vi "lab#5 (for loop).vi"() -> ()   [LabVIEW 2016]
panel:
  out "Elapsed Time (s)":dbl
  out "millisecond timer value":u32
  out "Time has Elapsed":bool
  out "number (0 to 1)":dbl
  out "Numeric 2":i32
  in  "Numeric":i32
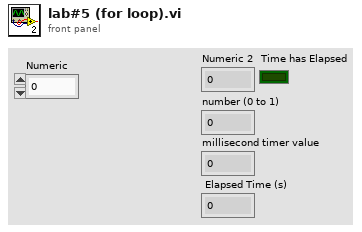
[diagram p1: front panel]
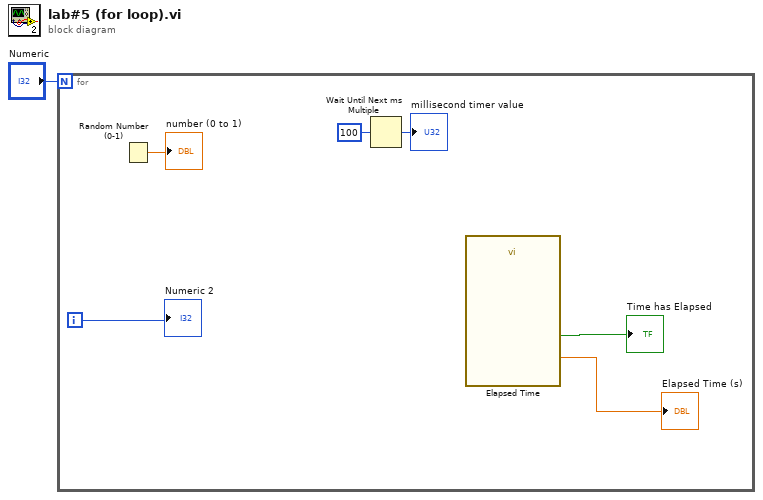
[diagram p0: block diagram]
diagram:
  n1 = for {
    N: "Numeric" -> [_]
    i -> [w7]
    n2 = Random Number (0-1)() -> (number: 0 to 1=→"number (0 to 1)":dbl)
    n3 = Wait Until Next ms Multiple(millisecond multiple=u32 100) -> (millisecond timer value=→"millisecond timer value":u32)
    n4 = call "Elapsed Time"() -> ("Elapsed Time (s)"=→"Elapsed Time (s)":dbl, "Time has Elapsed"=→"Time has Elapsed":bool)  [unwired: 12 in, 6 out]
    "Numeric 2" <- w7
  }
